vi "WPI_MotorControlRefNum Compare.vi"(1 "MotorControlDeviceRef 1":T1={"DeviceStatus"={"status"=FALSE, "code"=0, "source"=""}, "Type"=enum."PWM", "PWM"={"PWM Channel"=enum."Invalid", "DeadBand"={"Name"="", "maxPositivePwm"=0, "minPositivePwm"=0, "centerPwm"=0, "maxNegativePwm"=0, "minNegativePwm"=0, "angularRange"=0}}, "CAN"={"Device Number"=0, "SetOutput VI Ref"=variant(refnum<vi> refnum), "GetOutput VI Ref"=variant(refnum<vi> refnum), "Enable VI Ref"=variant(refnum<vi> refnum), "Disable VI Ref"=variant(refnum<vi> refnum), "Data"=variant}, "Invert"=FALSE, "DIO PWM"={"PWM \"Enable\" Channel"=enum."Invalid", "DIOChannel"=enum."Invalid", "PWM Rate"=0.0}}, 2 "MotorControlDeviceRef 2":T1={"DeviceStatus"={"status"=FALSE, "code"=0, "source"=""}, "Type"=enum."PWM", "PWM"={"PWM Channel"=enum."Invalid", "DeadBand"={"Name"="", "maxPositivePwm"=0, "minPositivePwm"=0, "centerPwm"=0, "maxNegativePwm"=0, "minNegativePwm"=0, "angularRange"=0}}, "CAN"={"Device Number"=0, "SetOutput VI Ref"=variant(refnum<vi> refnum), "GetOutput VI Ref"=variant(refnum<vi> refnum), "Enable VI Ref"=variant(refnum<vi> refnum), "Disable VI Ref"=variant(refnum<vi> refnum), "Data"=variant}, "Invert"=FALSE, "DIO PWM"={"PWM \"Enable\" Channel"=enum."Invalid", "DIOChannel"=enum."Invalid", "PWM Rate"=0.0}}) -> (5 "Equal?":bool)   [LabVIEW 2017]
uses:
  <vilib>/Rock Robotics/WPI/MotorControl/WPI_MotorControlDeviceRef.ctl
  <vilib>/Rock Robotics/WPI/MotorControl/WPI_MotorControlType.ctl
  <vilib>/Rock Robotics/SystemInterfaces/DIO/FPGA_DIOPWMChannel.ctl
  <vilib>/Rock Robotics/WPI/PWM/WPI_PWMDeadband.ctl
  <vilib>/Rock Robotics/SystemInterfaces/DIO/FPGA_DIOChannel.ctl
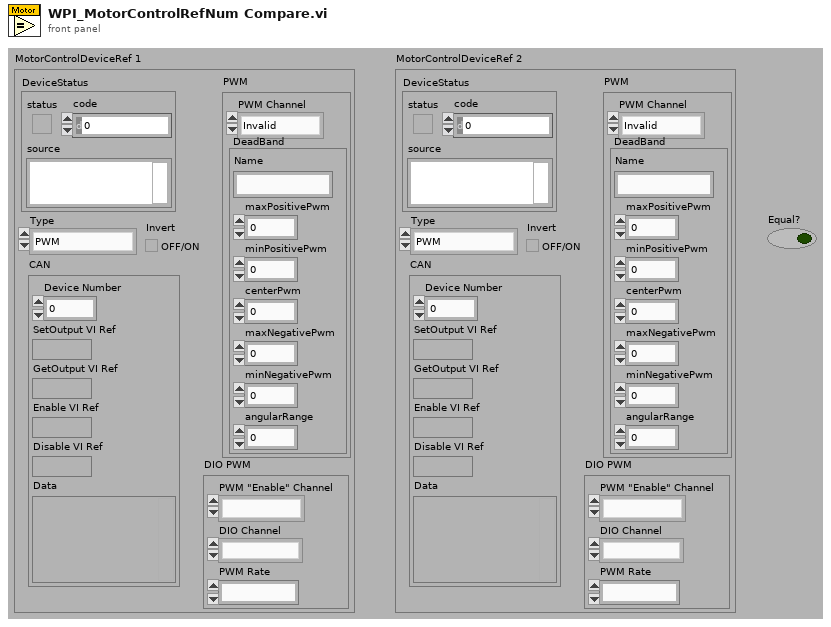
[diagram p1: front panel]
types:
  T1 = typedef "WPI_MotorControlDeviceRef.ctl" = cluster{"DeviceStatus":errorcluster, "Type":T2, "PWM":cluster{"PWM Channel":T3, "DeadBand":T4}, "CAN":cluster{"Device Number":u8, "SetOutput VI Ref":variant, "GetOutput VI Ref":variant, "Enable VI Ref":variant, "Disable VI Ref":variant, "Data":variant}, "Invert":bool, "DIO PWM":cluster{"PWM \"Enable\" Channel":T3, "DIOChannel":T5, "PWM Rate":dbl}}
  T2 = typedef "WPI_MotorControlType.ctl" = enum16{"PWM", "CAN", "DIO PWM"}
  T3 = typedef "FPGA_DIOPWMChannel.ctl" = enum8{"PWM 0", "PWM 1", "PWM 2", "PWM 3", "PWM 4", "PWM 5", "PWM 6", "PWM 7", "PWM 8", "PWM 9", "PWM MXP 0", "PWM MXP 1", "PWM MXP 2", "PWM MXP 3", "PWM MXP 4", "PWM MXP 5", "PWM MXP 6", "PWM MXP 7", "PWM MXP 8", "PWM MXP 9", "Invalid"}
  T4 = typedef "WPI_PWMDeadband.ctl" = cluster{"Name":string, "maxPositivePwm":i32, "minPositivePwm":i32, "centerPwm":i32, "maxNegativePwm":i32, "minNegativePwm":i32, "angularRange":u16}
  T5 = typedef "FPGA_DIOChannel.ctl" = enum8{"DIO 0", "DIO 1", "DIO 2", "DIO 3", "DIO 4", "DIO 5", "DIO 6", "DIO 7", "DIO 8", "DIO 9", "DIO MXP 0", "DIO MXP 1", "DIO MXP 2", "DIO MXP 3", "DIO MXP 4", "DIO MXP 5", "DIO MXP 6", "DIO MXP 7", "DIO MXP 8", "DIO MXP 9", "DIO MXP 10", "DIO MXP 11", "DIO MXP 12", "DIO MXP 13", "DIO MXP 14", "DIO MXP 15", "SPI Port CS1", "SPI Port CS2", "SPI Port CS3", "SPI Port MISO", "SPI Port MOSI", "Invalid"}
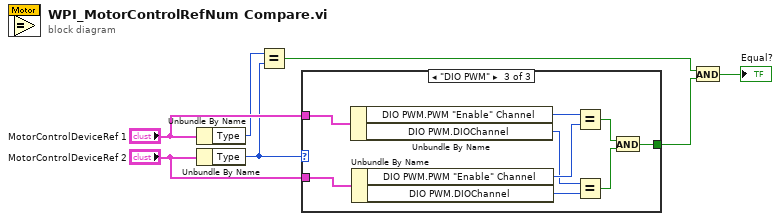
[diagram p0: block diagram]
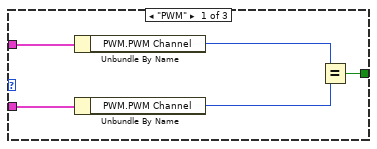
[diagram p2: hidden frame]
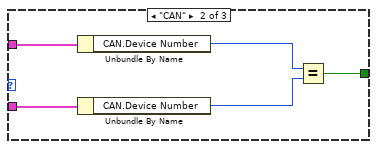
[diagram p3: hidden frame]
diagram:
  n1 = Unbundle By Name("MotorControlDeviceRef 1") -> ("Type"=w4:T2)
  n2 = Unbundle By Name("MotorControlDeviceRef 2") -> ("Type"=w5:T2)
  n3 = Equal?(x=w4, y=w5) -> (x = y?=w1:bool)
  n4 = case shown="\"DIO PWM\"" w5 {
    tunnel: "MotorControlDeviceRef 1" -> [w12 w17 w26]
    tunnel: "MotorControlDeviceRef 2" -> [w11 w16 w25]
    tunnel: [w10 w13 w19] -> w2
    frame "PWM" {
      n5 = Unbundle By Name(w12) -> ("PWM.PWM Channel"=w9:T3)
      n6 = Unbundle By Name(w11) -> ("PWM.PWM Channel"=w8:T3)
      n7 = Equal?(x=w9, y=w8) -> (x = y?=w10:bool)
    }
    frame "CAN" {
      n8 = Unbundle By Name(w17) -> ("CAN.Device Number"=w15:u8)
      n9 = Unbundle By Name(w16) -> ("CAN.Device Number"=w14:u8)
      n10 = Equal?(x=w15, y=w14) -> (x = y?=w13:bool)
    }
    frame "DIO PWM" {
      n11 = Unbundle By Name(w26) -> ("DIO PWM.PWM \"Enable\" Channel"=w24:T3, "DIO PWM.DIOChannel"=w21:T5)
      n12 = Unbundle By Name(w25) -> ("DIO PWM.PWM \"Enable\" Channel"=w23:T3, "DIO PWM.DIOChannel"=w20:T5)
      n13 = Equal?(x=w24, y=w23) -> (x = y?=w22:bool)
      n14 = Equal?(x=w21, y=w20) -> (x = y?=w18:bool)
      n15 = And(x=w22, y=w18) -> (x .and. y?=w19:bool)
    }
  }
  n16 = And(x=w1, y=w2) -> (x .and. y?=→"Equal?":bool)
